vi "Synchronized voice coil and stage signal.vi"() -> ()   [LabVIEW 2020]
uses:
  <vilib>/DAQmx/write.llb/DAQmx Write (Analog 1D Wfm NChan NSamp).vi
  <vilib>/DAQmx/create/channels.llb/DAQmx Create Channel (AO-Voltage-Basic).vi
  <vilib>/Analysis/1siggen.llb/Ramp Pattern by Delta.vi
  <vilib>/DAQmx/configure/timing.llb/DAQmx Timing (Use Waveform).vi
  <vilib>/DAQmx/miscellaneous.llb/DAQmx Fill In Error Info.vi
  <vilib>/Analysis/NI_AALBase.lvlib
panel:
  out "x/y":dbl
  out "samples":i32
  out "x*y":dbl
  out "Waveform Graph":waveform(dbl)[](graph)
  out "Square wave Graph":dbl[](graph)
  out "Sawtooth Graph":dbl[](graph)
  out "number of samples written per channel":u32
  out "Number of slices":dbl
  in  "End position (mm)":dbl
  out "Total Z thickness (mm)":dbl
  in  "Z slice width (mm)":dbl
  in  "Start position(mm)":dbl
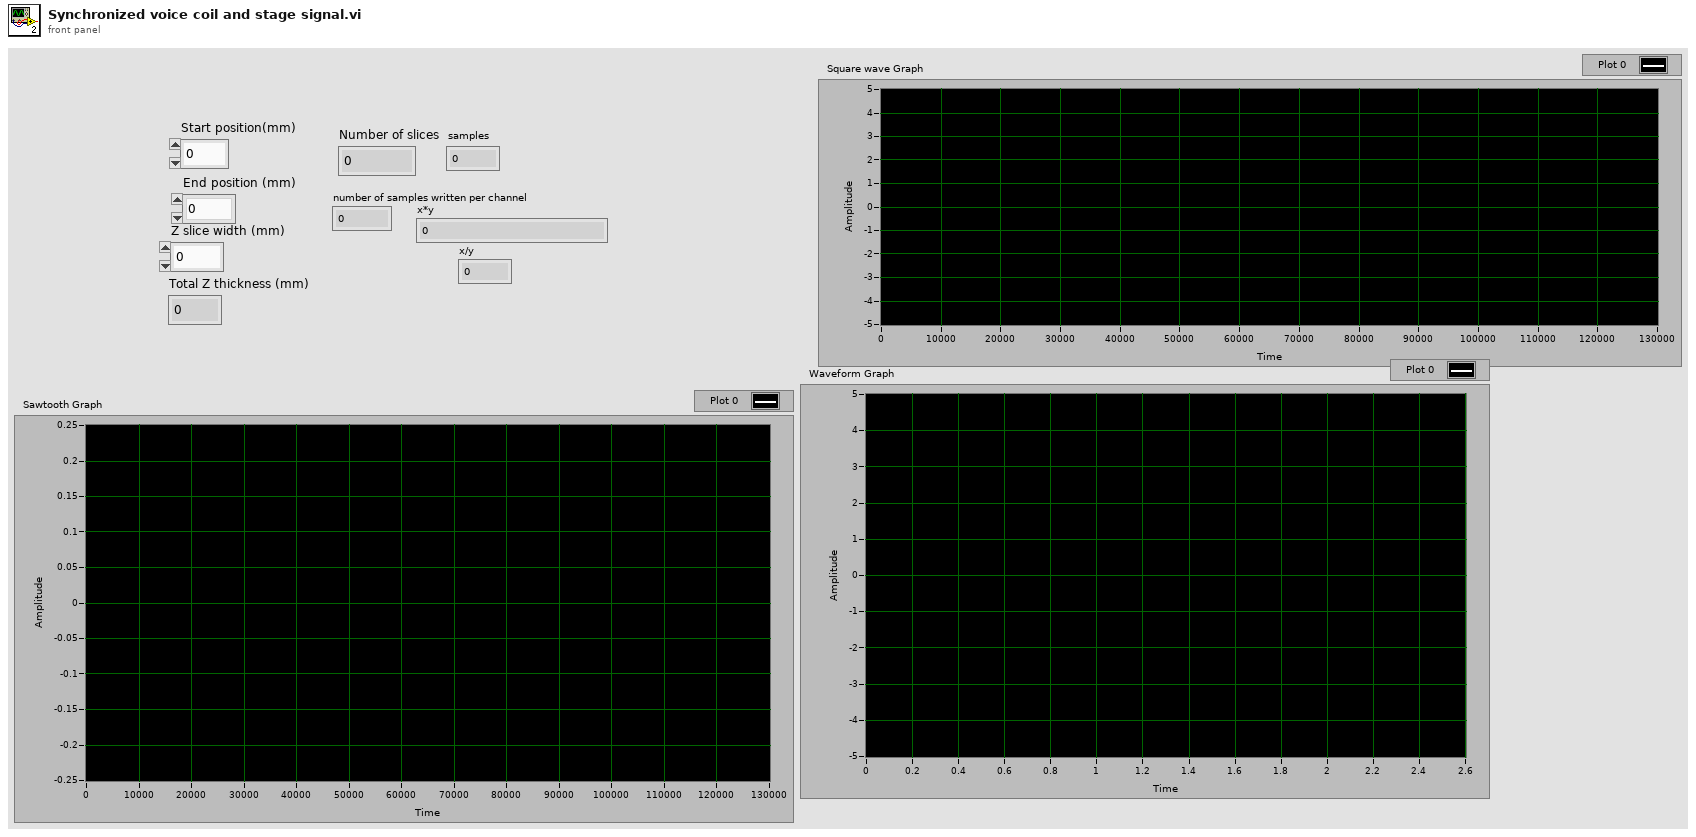
[diagram p1: front panel]
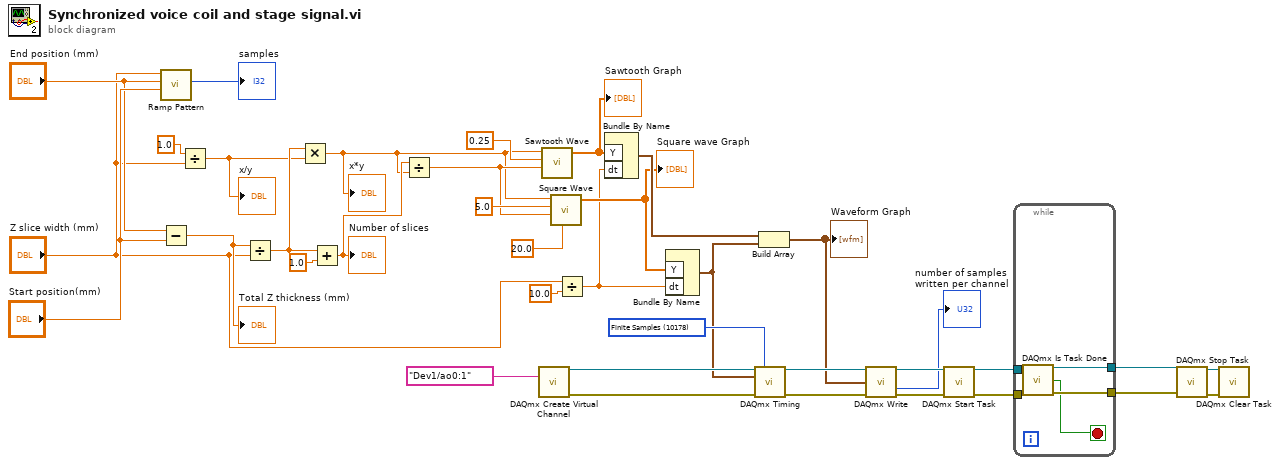
[diagram p0: block diagram]
diagram:
  w32 = 10178 items=["Finite Samples"=10178, "Continuous Samples"=10123, "Hardware Timed Single Point"=12522] ("sample mode")
  n1 = call-poly <vilib>:"Ramp Pattern.vi"("start"="Start position(mm)", "end"="End position (mm)", "delta"="Z slice width (mm)") -> ("samples"=→"samples":i32)  [unwired: 6 in, 2 out]
  n2 = Subtract(x="End position (mm)", y="Start position(mm)") -> (x-y=w21:dbl)
  "Total Z thickness (mm)" <- w21
  n3 = Divide(x=1.0, y="Z slice width (mm)") -> (x/y=w6:dbl)
  "x/y" <- w6
  n4 = Divide(x=w21, y="Z slice width (mm)") -> (x/y=w10:dbl)
  n5 = Multiply(x=w10, y=w6) -> (x*y=w5:dbl)
  "x*y" <- w5
  n6 = Add(x=w10, y=1.0) -> (x+y=w12:dbl)
  "Number of slices" <- w12
  n7 = Divide(x=w12, y=w5) -> (x/y=w11:dbl)
  n8 = call-poly <vilib>:"DAQmx Create Virtual Channel.vi"("physical channels"=tag "Dev1/ao0:1") -> ("task out"=w37:refnum<k21>, "error out"=w36:errorcluster)  [unwired: 13 in]
  n9 = call <vilib>:"Sawtooth Wave.vi"("samples"=w5, "amplitude"=0.25, "frequency"=w11) -> ("sawtooth wave"=w16:dbl[])  [unwired: 2 in, 2 out]
  "Sawtooth Graph" <- w16
  n10 = call <vilib>:"Square Wave.vi"("samples"=w5, "amplitude"=5.0, "frequency"=w11, "duty cycle (%)"=20.0) -> ("square wave"=w15:dbl[])  [unwired: 2 in, 2 out]
  "Square wave Graph" <- w15
  n11 = Divide(x="Z slice width (mm)", y=10.0) -> (x/y=w13:dbl)
  n12 = Bundle By Name("Y"=w16, "dt"=w13) -> (w22:waveform(dbl))  [unwired: 1 in]
  n13 = Bundle By Name("Y"=w15, "dt"=w13) -> (w9:waveform(dbl))  [unwired: 1 in]
  n14 = call-poly <vilib>:"DAQmx Timing.vi"("task/channels in"=w37, "sample mode"=w32, "waveform"=w9, "error in"=w36) -> ("task out"=w30:refnum<k21>, "error out"=w27:errorcluster)  [unwired: 10 in]
  n15 = Build Array(w22, w9) -> (w14:waveform(dbl)[])
  "Waveform Graph" <- w14
  n16 = call-poly <vilib>:"DAQmx Write.vi"("task/channels in"=w30, "data"=w14, "error in"=w27) -> ("task out"=w26:refnum<k21>, "number of samples written per channel"=→"number of samples written per channel":u32, "error out"=w25:errorcluster)  [unwired: 10 in]
  n17 = call <vilib>:"DAQmx Start Task.vi"("task/channels in"=w26, "error in"=w25) -> ("task out"=w4:refnum<k21>, "error out"=w3:errorcluster)  [unwired: 12 in]
  n18 = while {
    tunnel: w4 -> [w42]
    tunnel: w3 -> [w41]
    tunnel: [w40] -> w2
    tunnel: [w39] -> w1
    stop <- w38 stop-if-true
    n19 = call <vilib>:"DAQmx Is Task Done.vi"("task/channels in"=w42, "error in"=w41) -> ("task out"=w40:refnum<k21>, "task done?"=w38:bool, "error out"=w39:errorcluster)  [unwired: 11 in]
  }
  n20 = call <vilib>:"DAQmx Stop Task.vi"("task/channels in"=w2, "error in"=w1) -> ("task out"=w34:refnum<k21>, "error out"=w33:errorcluster)  [unwired: 12 in]
  n21 = call <vilib>:"DAQmx Clear Task.vi"("task in"=w34, "error in"=w33) -> ()  [unwired: 13 in, 1 out]
